vi "GA Set Jog Prm Single.vi"(7 "dSmooth":dbl, 8 "error in (no error)":errorcluster caption="错误输入（无错误）", 9 "dDec":dbl, 10 "dAcc":dbl, 11 "nAxisNum":i16) -> (0 "error out":errorcluster caption="错误输出", 3 "function return":i32)   [LabVIEW 2015, in "GAS.lvlib"]
doc: "extern \"C\" __declspec(dllimport) int GA_SetJogPrmSingle(short nAxisNum,double dAcc,double dDec,double dSmooth);"
uses:
  <userlib>/BP_GAS/GAS.lvlib
  <userlib>/BP_GAS/GAS.dll
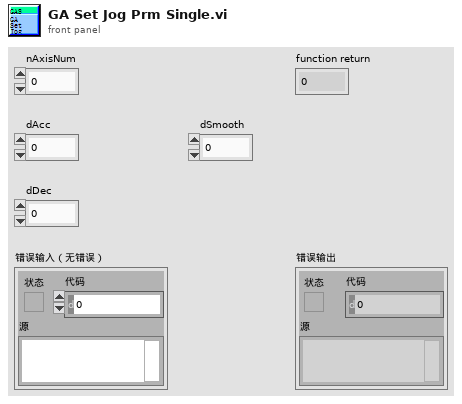
[diagram p1: front panel]
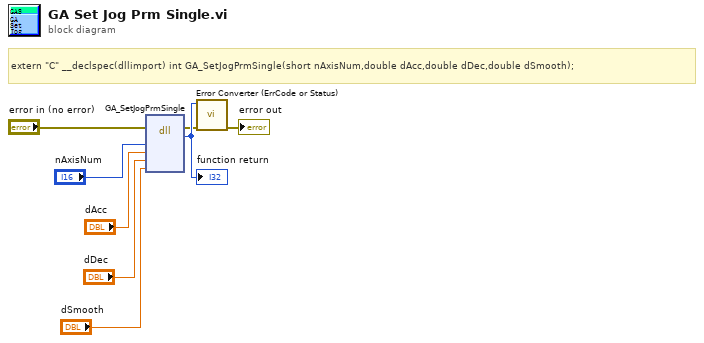
[diagram p0: block diagram]
diagram:
  # "extern \"C\" __declspec(dllimport) int GA_SetJogPrmSingle(short nAxisNum,double dAcc,double dDec,double dSmooth);"
  n1 = dll-call lib="E:/Program Files (x86)/National Instruments/LabVIEW 2015/user.lib/BP_GAS/GAS.*" fn="GA_SetJogPrmSingle"(error in="error in (no error)", "nAxisNum"="nAxisNum", "dAcc"="dAcc", "dDec"="dDec", "dSmooth"="dSmooth") -> (error out=w2:errorcluster, w8:i32)  [unwired: 6 in, 1 out]
  "function return" <- w8
  n2 = call "Error Converter (ErrCode or Status).vi"("error in (no error)"=w2, "error code"=w8) -> ("error out"=→"error out":errorcluster)  [unwired: 9 in]
